vi "SortVoltage_Display.vi"(10 "Voltage":T1={"TimeString"="", "Time Stamp"=0.0, "AI0_Unused"=0.033825768742891164, "AI1_-5V"=0.03350358521901454, "AI2_+5V"=0.03414795226674084, "AI3_+6V"=-0.0003256849402108635, "AI4_+12V"=-0.0012922355206829907, "AI5_+15V"=-0.0012922355206829907, "AI6_+28V"=-0.020301063655153495, "AI7_Unused"=-0.0006478684670067779, "Ai16_72GHz_CalPower"=-0.0022587861014084333, "Ai17_84GHz_CalPower"=-0.0038697037365145624, "Ai18_InclinAz"=-0.0966585607532968, "Ai19_InclinEl"=-0.09698074428898816, "Ai20_BlowerPwr"=-0.10890153513172597, "Ai21_Unused"=-0.09891384550379581, "Ai22_Unused"=-0.11663394002592792, "Ai23_Unused"=-0.0009700519938308167, "InclinA_StdDev"=0.0, "InclinB_StdDev"=0.0, "InclinAz_Unfilt"=0.0, "InclinEl_Unfilt"=0.0} {"Ai23_Unused" format="%#.2g"; "Ai22_Unused" format="%#.2g"; "Ai21_Unused" format="%#.2g"; "Ai20_BlowerPwr" format="%#.2g"; "Ai19_InclinEl" format="%#.2g"; "Ai18_InclinAz" format="%#.2g"; "Ai17_84GHz_CalPower" format="%#.2g"; "Ai16_72GHz_CalPower" format="%#.2g"; "AI7_Unused" format="%#.2g"; "AI6_+28V" format="%#.2g"; "AI5_+15V" format="%#.2g"; "AI4_+12V" format="%#.2g"; "AI3_+6V" format="%#.2g"; "AI2_+5V" format="%#.2g"; "AI1_-5V" format="%#.2g"; "AI0_Unused" format="%#.2g"}) -> (2 "VoltageDisplay":T2={"AI0_Unused"=0.033825768742891164, "AI1_-5V"=0.03350358521901454, "AI2_+5V"=0.03414795226674084, "AI3_+6V"=-0.0003256849402108635, "AI4_+12V"=-0.0012922355206829907, "AI5_+15V"=-0.0012922355206829907, "AI6_+28V"=-0.020301063655153495, "Ai16_72GHz_CalPower"=-0.0022587861014084333, "Ai17_84GHz_CalPower"=-0.0038697037365145624, "Ai18_InclinometerAz"=-0.0038697037365145624, "Ai19_InclinometerEl"=-0.0038697037365145624, "Az_StdDev"=-0.0038697037365145624, "El_StdDev"=-0.0038697037365145624, "Ai20_BlowerPower"=-0.0038697037365145624} {"Ai20_BlowerPower" format="%#.2g"; "El_StdDev" format="%#.2g"; "Az_StdDev" format="%#.2g"; "Ai19_InclinometerEl" format="%#.2g"; "Ai18_InclinometerAz" format="%#.2g"; "Ai17_84GHz_CalPower" format="%#.2g"; "Ai16_72GHz_CalPower" format="%#.2g"; "AI6_+28V" format="%#.2g"; "AI5_+15V" format="%#.2g"; "AI4_+12V" format="%#.2g"; "AI3_+6V" format="%#.2g"; "AI2_+5V" format="%#.2g"; "AI1_-5V" format="%#.2g"; "AI0_Unused" format="%#.2g"})   [LabVIEW 2018]
uses:
  Controls/Clusts/Voltage_Display_Clust.ctl
  Controls/Clusts/AI_Clust.ctl
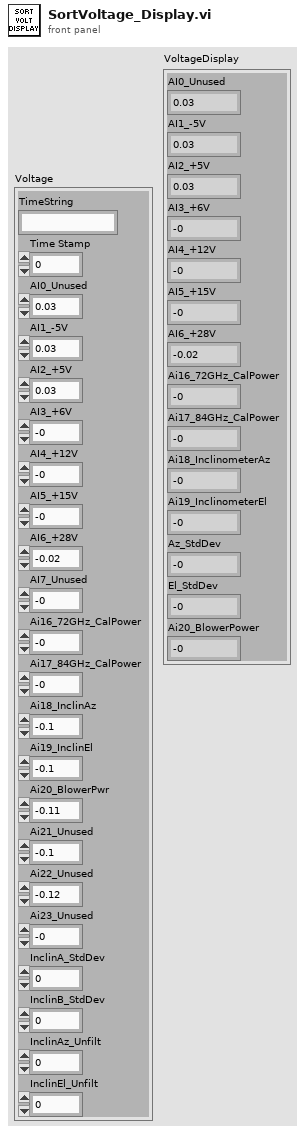
[diagram p1: front panel]
types:
  T1 = typedef "AI_Clust.ctl" = cluster{"TimeString":string, "Time Stamp":dbl, "AI0_Unused":dbl, "AI1_-5V":dbl, "AI2_+5V":dbl, "AI3_+6V":dbl, "AI4_+12V":dbl, "AI5_+15V":dbl, "AI6_+28V":dbl, "AI7_Unused":dbl, "Ai16_72GHz_CalPower":dbl, "Ai17_84GHz_CalPower":dbl, "Ai18_InclinAz":dbl, "Ai19_InclinEl":dbl, "Ai20_BlowerPwr":dbl, "Ai21_Unused":dbl, "Ai22_Unused":dbl, "Ai23_Unused":dbl, "InclinA_StdDev":dbl, "InclinB_StdDev":dbl, "InclinAz_Unfilt":dbl, "InclinEl_Unfilt":dbl}
  T2 = typedef "Voltage_Display_Clust.ctl" = cluster{"AI0_Unused":dbl, "AI1_-5V":dbl, "AI2_+5V":dbl, "AI3_+6V":dbl, "AI4_+12V":dbl, "AI5_+15V":dbl, "AI6_+28V":dbl, "Ai16_72GHz_CalPower":dbl, "Ai17_84GHz_CalPower":dbl, "Ai18_InclinometerAz":dbl, "Ai19_InclinometerEl":dbl, "Az_StdDev":dbl, "El_StdDev":dbl, "Ai20_BlowerPower":dbl}
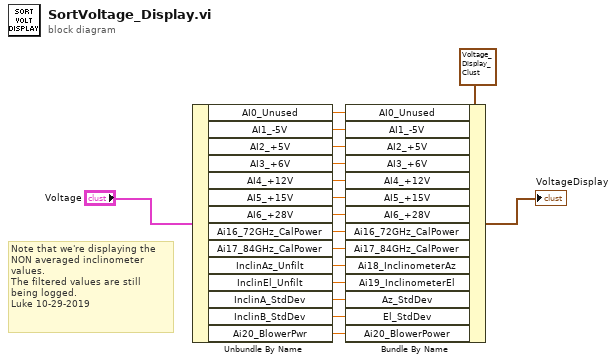
[diagram p0: block diagram]
diagram:
  # "Note that we're displaying the \nNON averaged inclinometer\nvalues.\nThe filtered values are still\nbeing logged.\nLuke 10-29-2019"
  n1 = Unbundle By Name("Voltage") -> ("AI0_Unused"=w9:dbl, "AI1_-5V"=w10:dbl, "AI2_+5V"=w11:dbl, "AI3_+6V"=w12:dbl, "AI4_+12V"=w13:dbl, "AI5_+15V"=w14:dbl, "AI6_+28V"=w15:dbl, "Ai16_72GHz_CalPower"=w16:dbl, "Ai17_84GHz_CalPower"=w17:dbl, "InclinAz_Unfilt"=w5:dbl, "InclinEl_Unfilt"=w4:dbl, "InclinA_StdDev"=w3:dbl, "InclinB_StdDev"=w2:dbl, "Ai20_BlowerPwr"=w1:dbl)
  n2 = Bundle By Name(cluster=T2 {"AI0_Unused"=0.033825768742891164, "AI1_-5V"=0.03350358521901454, "AI2_+5V"=0.03414795226674084, "AI3_+6V"=-0.0003256849402108635, "AI4_+12V"=-0.0012922355206829907, "AI5_+15V"=-0.0012922355206829907, "AI6_+28V"=-0.020301063655153495, "Ai16_72GHz_CalPower"=-0.0022587861014084333, "Ai17_84GHz_CalPower"=-0.0038697037365145624, "Ai18_InclinometerAz"=-0.0038697037365145624, "Ai19_InclinometerEl"=-0.0038697037365145624, "Az_StdDev"=-0.0038697037365145624, "El_StdDev"=-0.0038697037365145624, "Ai20_BlowerPower"=-0.0038697037365145624} ("VoltageDisplay 2"), "AI0_Unused"=w9, "AI1_-5V"=w10, "AI2_+5V"=w11, "AI3_+6V"=w12, "AI4_+12V"=w13, "AI5_+15V"=w14, "AI6_+28V"=w15, "Ai16_72GHz_CalPower"=w16, "Ai17_84GHz_CalPower"=w17, "Ai18_InclinometerAz"=w5, "Ai19_InclinometerEl"=w4, "Az_StdDev"=w3, "El_StdDev"=w2, "Ai20_BlowerPower"=w1) -> (→"VoltageDisplay":T2)
